vi "Factory Core.vi"(8 "error in (no error)":errorcluster, 11 "Protocol Interface in":refnum<class "Protocol Interface.lvclass">) -> (0 "error out":errorcluster, 3 "Protocol Interface out":refnum<class "Protocol Interface.lvclass">)   [LabVIEW 2018, in "Protocol Interface.lvlib" / "Protocol Interface.lvclass"]
uses:
  Protocol Interface.lvclass
  FPF.lvlibp/Factory Plugin Framework.lvclass
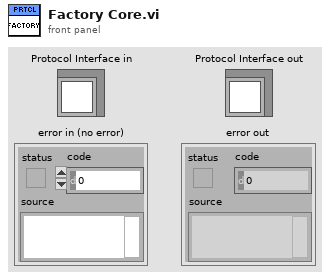
[diagram p1: front panel]
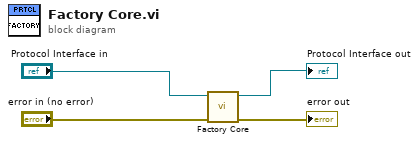
[diagram p0: block diagram]
diagram:
  n1 = call-parent "Factory Core.vi"("error in (no error)"="error in (no error)", "Factory Plugin Framework in"="Protocol Interface in") -> ("error out"=→"error out":errorcluster, "Factory Plugin Framework out"=→"Protocol Interface out":refnum<class "Protocol Interface.lvclass">)  [unwired: 8 in]
